vi "Arbitrary Wave Display.vi"() -> ()   [LabVIEW 2023]
doc: "This VI demonstrates the use of the Arbitrary Wave signal generator VI. The top waveform graph shows the arbitrary wave array generated using the input controls. The diagram shows how to convert from these common frequency units to the \"normalized\" frequency units of cycles/sample (cycles/sample is the unit used by the Sine Wave, Triangle Wave, Square Wave, Sawtooth Wave, Arbitrary Wave, and Chirp Pattern VIs.) The Waveform Pattern simply plots the points given in the input array Wave Table, which represents 1 cycle of the arbitrary wave. If reset phase is set to OFF (false), the Arbitrary Wave VI will output the next samples of the waveform, preserving a continuously smooth phase."
uses:
  <vilib>/Analysis/NI_AALBase.lvlib
panel:
  in  "Frequency Unit":u16(ring) items=["Hz", "cycles"]
  in  "Stop":bool
  in  "Reset phase":bool
  in  "Sampling rate (Hz)":dbl=100.0 step=1.0 format="%#.3g"
  out "Waveform Pattern":dbl[](graph)
  out "Signal Generated":T1(graph)={0.0, 0.01, "arbitrary wave"=[]}
  in  "interpolation":i32(ring)=1 items=["none", "linear"]
  in  "Wave Table":dbl[](array[numeric])=[0.0, 1.0, 4.0, 0.2, -0.9]
  in  "Frequency":dbl=2.01 step=1.0 format="%0.2f"
  in  "Amplitude":dbl(slide)=3.7755102040816326 scale=0.0..5.0
  # "Overview: Demonstrates the use of the Arbitrary Wave VI.\nRequirements: LabVIEW Full Development System\nInstructions: \n1. Run the VI.\n2. Adjust the Frequency and interpolation method.  \n3. Edit a single cycle of the arbitrary waveform by changing the Wave Table array, plotted in the Waveform Pattern graph. \n4. Click Stop to stop the VI."
  # "Signal Generation Parameters"
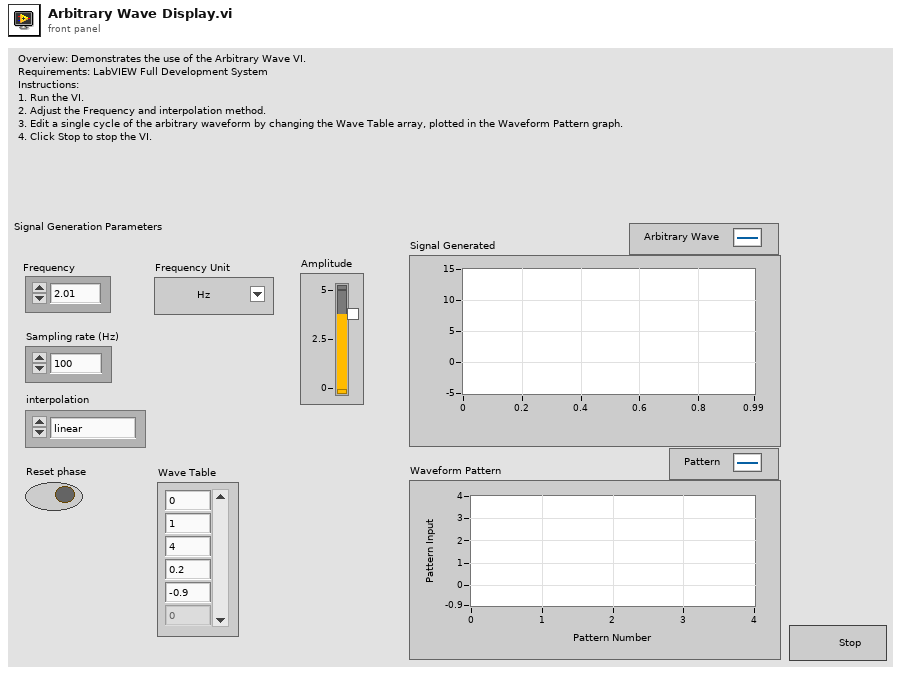
[diagram p1: front panel]
types:
  T1 = cluster{dbl[unit], dbl[unit], "arbitrary wave":dbl[]}
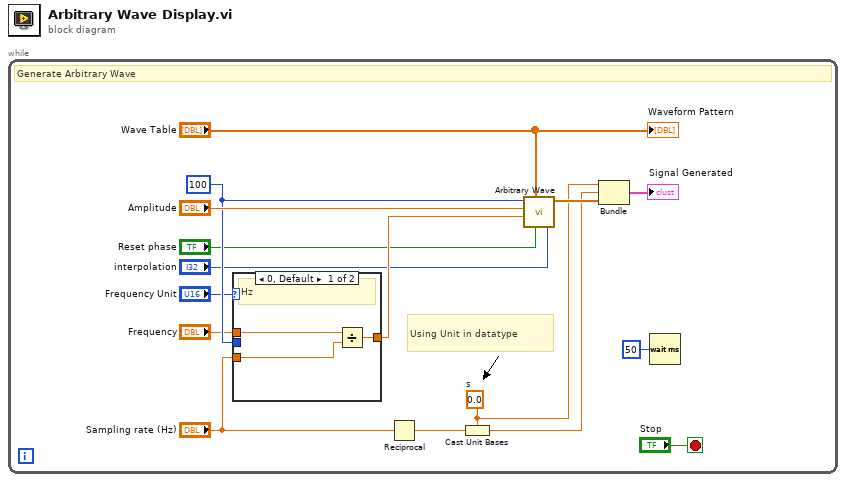
[diagram p0: block diagram]
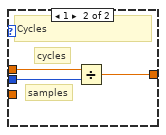
[diagram p2: hidden frame]
diagram:
  n1 = while {
    stop <- "Stop" stop-if-true
    w2 = dbl[unit] 0.0  # s
    w13 = 100 ("samples")
    # "Using Unit in datatype"
    # "Generate Arbitrary Wave"
    n2 = case shown="0, Default" "Frequency Unit" {
      tunnel: [w19 w21] -> w14
      tunnel: w13 -> [_ w22]
      tunnel: "Frequency" -> [w18 w20]
      tunnel: "Sampling rate (Hz)" -> [w17 _]
      frame 0, Default {
        # "Hz"
        n3 = Divide(x=w18, y=w17) -> (x/y=w19:dbl)
      }
      frame 1 {
        # "samples"
        # "cycles"
        # "Cycles"
        n4 = Divide(x=w20, y=w22) -> (x/y=w21:dbl)
      }
    }
    n5 = Reciprocal(x="Sampling rate (Hz)") -> (1/x=w7:dbl)
    n6 = Cast Unit Bases(0:w7, 1:w2) -> (2:w6:dbl[unit])
    n7 = call <vilib>:"Arbitrary Wave.vi"("interpolation"="interpolation", "reset phase"="Reset phase", "Wave Table"="Wave Table", "frequency"=w14, "amplitude"="Amplitude", "samples"=w13) -> ("arbitrary wave"=w9:dbl[])  [unwired: 1 in, 2 out]
    n8 = Bundle(w2, w6, "arbitrary wave"=w9) -> (→"Signal Generated":T1)  [unwired: 1 in]
    n9 = Wait (ms)(milliseconds to wait=u32 50) -> ()  [unwired: 1 out]
    "Waveform Pattern" <- "Wave Table"
  }
